vi "Read Register.vi"(0 "Refnum in":refnum<visa-resource-name>, 5 "Mode":T2, 7 "startReg":u16, 9 "Quantity":u16=1, 11 "error in (no error)":errorcluster) -> (4 "Refnum Out":refnum<visa-resource-name>, 6 "ModeOut":T1, 8 "Holding Registers":u16[](array[numeric]), 10 "Numeric":i16, 15 "error out":errorcluster)   [LabVIEW 2020]
uses:
  <vilib>/NI Modbus.llb/MB Serial Master Query Read Holding Registers (poly).vi
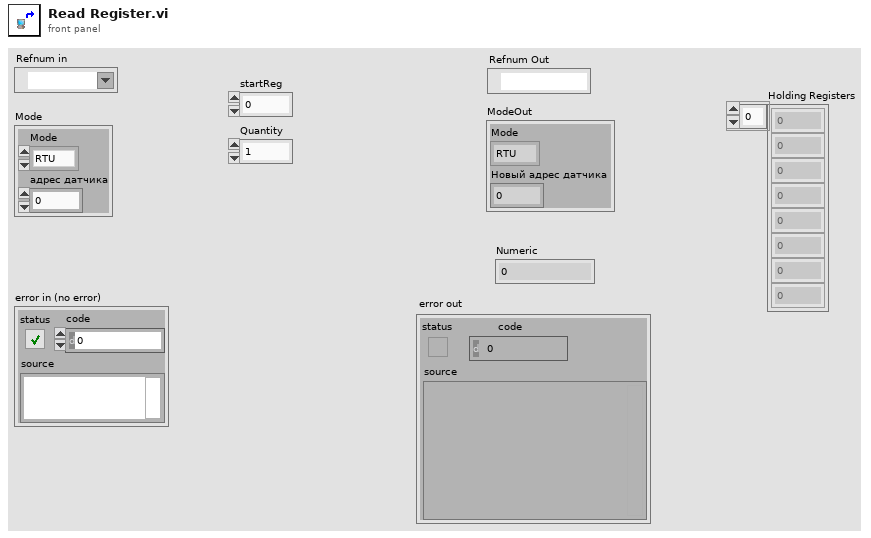
[diagram p1: front panel]
types:
  T1 = cluster{"Mode":enum16{"RTU", "ASCII"}, "Новый адрес датчика":u16}
  T2 = cluster{"Mode":enum16{"RTU", "ASCII"}, "адрес датчика":u16}
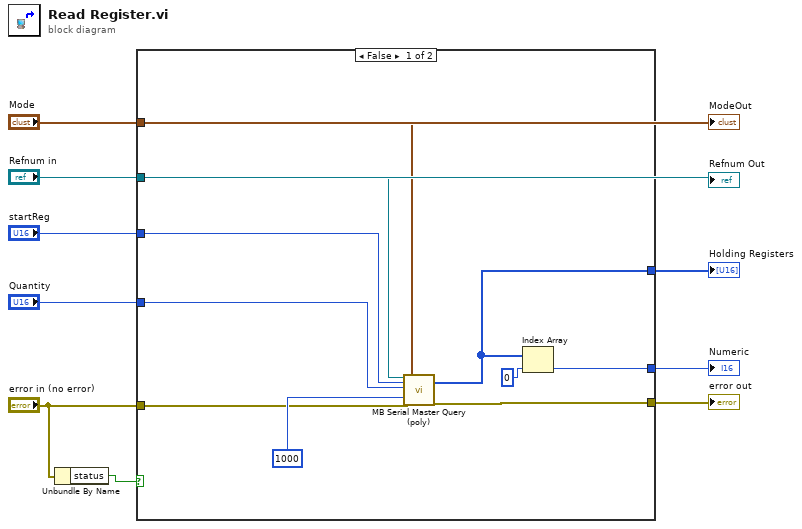
[diagram p0: block diagram]
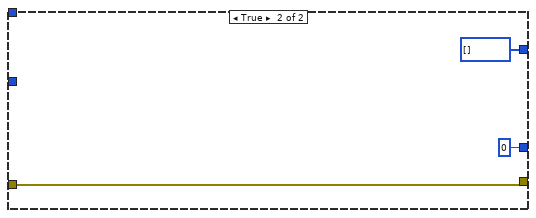
[diagram p2: hidden frame]
diagram:
  n1 = Unbundle By Name("error in (no error)") -> ("status"=w1:bool)
  n2 = case shown="False" w1 {
    tunnel: [w18 u16[] [] ("Holding Registers")] -> w9
    tunnel: "Mode" -> [w16 _]
    tunnel: "error in (no error)" -> [w15 w22]
    tunnel: "Refnum in" -> [w14 _]
    tunnel: "startReg" -> [w13 _]
    tunnel: "Quantity" -> [w12 _]
    tunnel: [w11 u16 0 ("Numeric")] -> w4
    tunnel: [w10 w22] -> w3
    frame False {
      n3 = call-poly <vilib>:"MB Serial Master Query (poly).vi"("VISA resource name"=w14, "Starting Address"=w13, "Quantity"=w12, "Timeout"=u32 1000, "error in"=w15, "Serial Parameters"=w16) -> ("Holding Registers"=w18:u16[], "error out"=w10:errorcluster)  [unwired: 12 out]
      n4 = Index Array(array=w18, index=u16 0 ("Starting Address")) -> (element=w11:u16)
    }
    frame True {
    }
  }
  "Numeric" <- w4
  "error out" <- w3
  "Holding Registers" <- w9
  "ModeOut" <- "Mode"
  "Refnum Out" <- "Refnum in"
